vi "HalfAdderCircuit.vi"() -> ()   [LabVIEW 2019]
panel:
  out "Carry":bool
  out "SUM":bool
  in  "Input Two":bool
  in  "Input One":bool
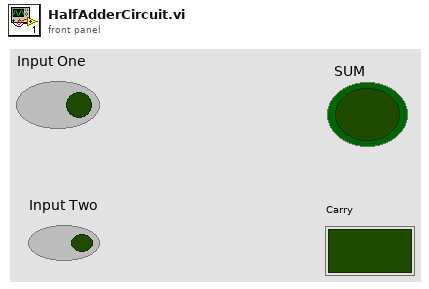
[diagram p1: front panel]
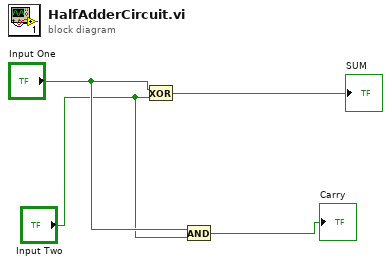
[diagram p0: block diagram]
diagram:
  n1 = Exclusive Or(1:"Input Two", 2:"Input One") -> (0:→"SUM":bool)
  n2 = And(x="Input One", y="Input Two") -> (x .and. y?=→"Carry":bool)
